vi "grab aoi.vi"(10 "Ccd No.":enum16{"non", "glue ccd", "alone ccd"}(ring), 11 "引用句柄输入":T1) -> (3 "引用句柄输出":T1)   [LabVIEW 2015]
uses:
  <vilib>/vision/Image Controls.llb/IMAQ Image.ctl
  <vilib>/userdefined/High Color/IMAQdx.ctl
  <vilib>/vision/driver/NI_Vision_Acquisition_Software.lvlib
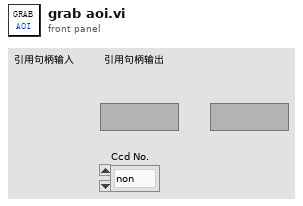
[diagram p1: front panel]
types:
  T1 = typedef "IMAQ Image.ctl" = refnum<image>
  T2 = typedef "IMAQdx.ctl" = refnum<k21>
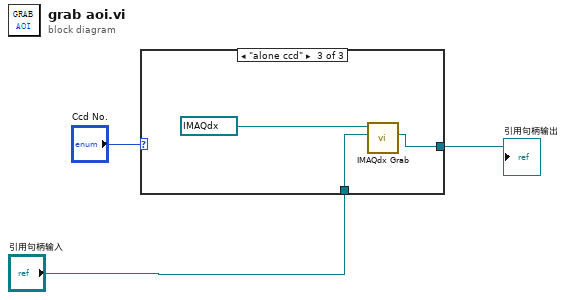
[diagram p0: block diagram]
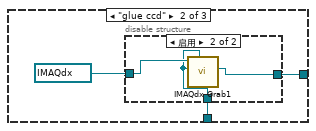
[diagram p3: hidden frame]
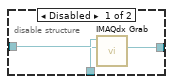
[diagram p4: hidden frame]
diagram:
  n1 = case shown="\"alone ccd\"" "Ccd No." {
    tunnel: "引用句柄输入" -> [w4 w6 w15]
    tunnel: [w4 w5 w14] -> w3
    frame "non", Default {
      # "readpic"
    }
    frame "glue ccd" {
      n2 = disable-structure shown="启用" {
        disable-tunnel: T2 "cam0" ("Session In") -> [w10 w13]
        disable-tunnel: w6 -> [w9 w11]
        disable-tunnel: [w8 w12] -> w5
        frame Disabled {
          n3 = call <vilib>:"IMAQdx Grab.vi"("Image In"=w9, "Session In"=w10) -> ("Image Out"=w8:T1)  [unwired: 6 in, 3 out]
        }
        frame Enabled {
          n4 = call "IMAQdx Grab1.vi"("New Image"=w11, "Image In"=w11, "Session In"=w13) -> ("Image Out"=w12:T1)  [unwired: 5 in, 3 out]
        }
      }
    }
    frame "alone ccd" {
      n5 = call <vilib>:"IMAQdx Grab.vi"("Image In"=w15, "Session In"=T2 "cam1") -> ("Image Out"=w14:T1)  [unwired: 6 in, 3 out]
    }
  }
  "引用句柄输出" <- w3
